vi "uTTA_GetDeviceCalibration.vi"(4 "error in":errorcluster, 7 "VISA Refnum in":refnum<visa-resource-name>) -> (0 "error out":errorcluster, 1 "uTTA_CalData":T1(array[cluster]), 2 "Received":string, 3 "VISA Refnum out":refnum<visa-resource-name>)   [LabVIEW 2021]
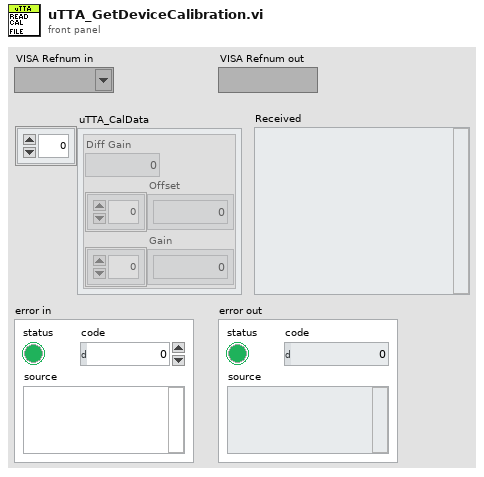
[diagram p1: front panel]
types:
  T1 = cluster{"Diff Gain":dbl, "Offset":dbl[], "Gain":dbl[]}[]
  T2 = cluster{"Diff Gain":dbl, "Offset":dbl[], "Gain":dbl[]}
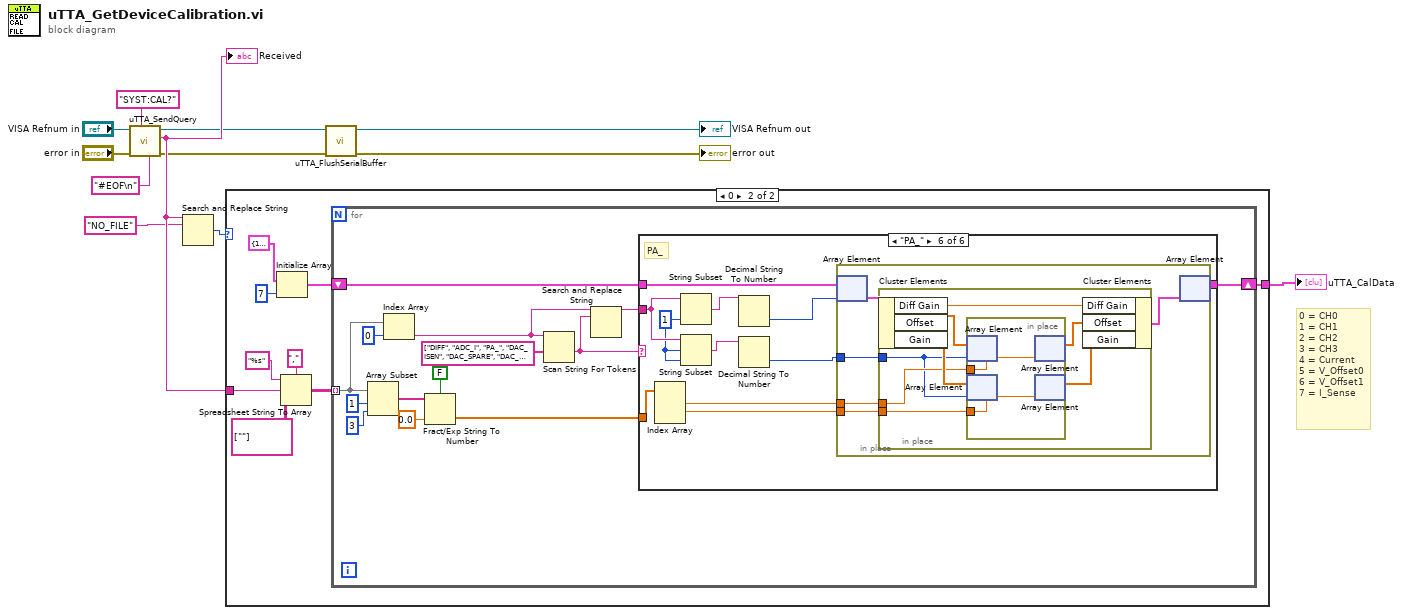
[diagram p0: block diagram]
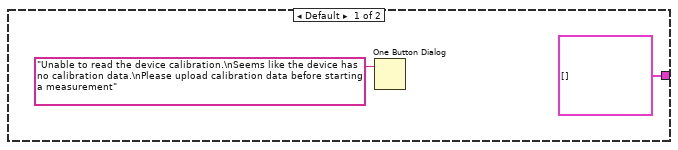
[diagram p2: hidden frame]
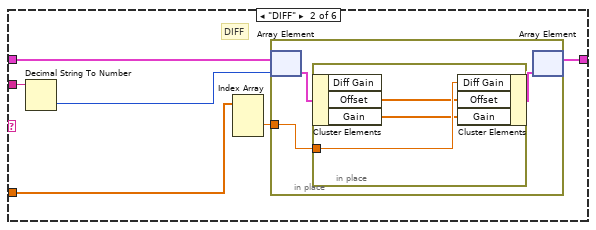
[diagram p4: hidden frame]
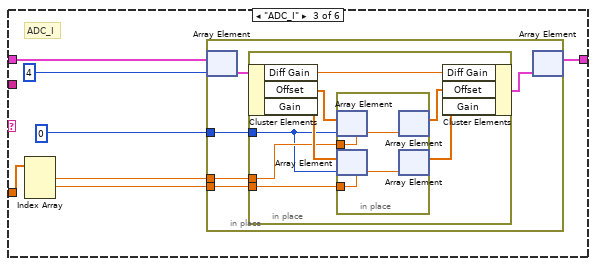
[diagram p5: hidden frame]
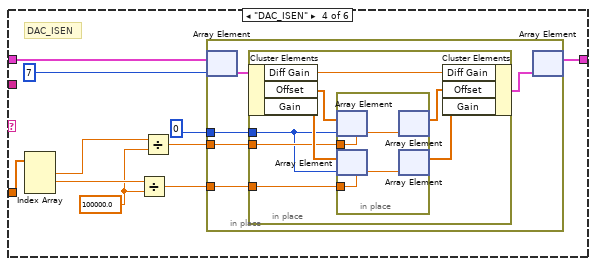
[diagram p6: hidden frame]
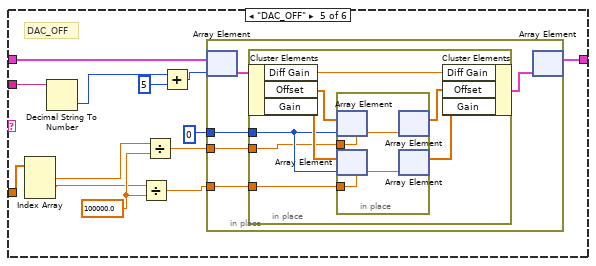
[diagram p7: hidden frame]
diagram:
  # "0 = CH0\n1 = CH1\n2 = CH2\n3 = CH3\n4 = Current\n5 = V_Offset0\n6 = V_Offset1\n7 = I_Sense"
  n1 = call "uTTA_SendQuery.vi"("RX Termination(\\n)"="#EOF\n" ("RX Termination(\\n)"), "Send String"="SYST:CAL?", "error in (no error)"="error in", "VISA Refnum in"="VISA Refnum in") -> ("error out"=w5:errorcluster, "Received"=w8:string, "VISA Refnum out"=w4:refnum<visa-resource-name>)  [unwired: 5 in]
  "Received" <- w8
  n2 = Search and Replace String(input string=w8, search string="NO_FILE") -> (number of replacements=w6:i32)  [unwired: 6 in, 3 out]
  n3 = case shown="0" w6 {
    tunnel: [T1 [] w17] -> w9
    tunnel: w8 -> [_ w16]
    frame Default {
      n4 = One Button Dialog(message="Unable to read the device calibration.\nSeems like the device has no calibration data.\nPlease upload calibration data before starting a measurement") -> ()  [unwired: 1 in, 1 out]
    }
    frame 0 {
      n5 = Initialize Array(T2 {"Diff Gain"=1.0, "Offset"=[0.0, 0.0, 0.0, 0.0], "Gain"=[0.0, 0.0, 0.0, 0.0]} ("Cluster"), 7 ("dimension size")) -> (w18:T1)
      n6 = Spreadsheet String To Array(delimiter (Tab)=",", format string="%s", spreadsheet string=w16, array type (2D Dbl)=string[][] [[""]]) -> (array=w21:string[][])
      n7 = for {
        tunnel: w21 -> [w34] mode=indexing
        shift-right: [w35] -> w17
        shift-left: w18 -> [w36]
        n8 = Array Subset(array=w34, index=1, length=3) -> (w31:string[])
        n9 = Index Array(array=w34, index=0) -> (element=w26:string)
        n10 = Fract/Exp String To Number(use system decimal point (T)=FALSE, string=w31, default (0 dbl)=0.0 ("default (0 DBL)")) -> (number=w28:dbl[])  [unwired: 1 in, 1 out]
        n11 = Scan String For Tokens(7:string[] ["DIFF", "ADC_I", "PA_", "DAC_ISEN", "DAC_SPARE", "DAC_OFF"] ("operators (none)"), 9:w26) -> (1:w25:string)  [unwired: 4 in, 3 out]
        n12 = Search and Replace String(input string=w26, search string=w25) -> (result string=w24:string)  [unwired: 6 in, 3 out]
        n13 = case shown="\"PA_\"" w25 {
          tunnel: w36 -> [w38 w44 w56 w81 w110 w136]
          tunnel: [w38 w43 w55 w80 w109 w135] -> w35
          tunnel: w28 -> [_ w42 w54 w79 w108 w134]
          tunnel: w24 -> [_ w40 _ _ w106 w131]
          frame Default {
          }
          frame "DIFF" {
            # "DIFF"
            n14 = Decimal String To Number(string=w40) -> (number=w39:i32)  [unwired: 2 in, 1 out]
            n15 = Index Array(array=w42) -> (element #2=w41:dbl)  [unwired: 3 in, 2 out]
            n16 = in-place {
              in-place-border: w41 -> [w45]
              n17 = in-place-array #1(w44, w39) -> (w47:T2)
              n18 = in-place {
                in-place-border: w45 -> [w50]
                n19 = in-place-cluster #2(w47) -> ("Offset"=w49:dbl[], "Gain"=w48:dbl[])  [unwired: 1 out]
                n20 = in-place-cluster #2("Diff Gain"=w50, "Offset"=w49, "Gain"=w48) -> (w46:T2)
              }
              n21 = in-place-array #1(w46) -> (w43:T1)  [unwired: 1 out]
            }
          }
          frame "ADC_I" {
            # "ADC_I"
            n22 = Index Array(array=w54) -> (element #1=w52:dbl, element #2=w53:dbl)  [unwired: 3 in, 1 out]
            n23 = in-place {
              in-place-border: w53 -> [w60]
              in-place-border: w52 -> [w59]
              in-place-border: 0 -> [w58]
              n24 = in-place-array #3(w56, 4) -> (w62:T2)
              n25 = in-place {
                in-place-border: w60 -> [w65]
                in-place-border: w59 -> [w66]
                in-place-border: w58 -> [w64]
                n26 = in-place-cluster #4(w62) -> ("Diff Gain"=w63:dbl, "Offset"=w70:dbl[], "Gain"=w69:dbl[])
                n27 = in-place {
                  in-place-border: w66 -> [w72]
                  in-place-border: w65 -> [w71]
                  n28 = in-place-array #5(w70, w64) -> ()  [unwired: 1 out]
                  n29 = in-place-array #6(w69, w64) -> ()  [unwired: 1 out]
                  n30 = in-place-array #5(w72) -> (w68:dbl[])  [unwired: 1 out]
                  n31 = in-place-array #6(w71) -> (w67:dbl[])  [unwired: 1 out]
                }
                n32 = in-place-cluster #4("Diff Gain"=w63, "Offset"=w68, "Gain"=w67) -> (w61:T2)
              }
              n33 = in-place-array #3(w61) -> (w55:T1)  [unwired: 1 out]
            }
          }
          frame "DAC_ISEN" {
            w73 = 100000.0 ("y")
            # "DAC_ISEN"
            n34 = Index Array(array=w79) -> (element #1=w77:dbl, element #2=w75:dbl)  [unwired: 3 in, 1 out]
            n35 = Divide(x=w75, y=w73) -> (x/y=w74:dbl)
            n36 = Divide(x=w77, y=w73) -> (x/y=w76:dbl)
            n37 = in-place {
              in-place-border: w74 -> [w85]
              in-place-border: w76 -> [w84]
              in-place-border: 0 -> [w83]
              n38 = in-place-array #7(w81, 7) -> (w87:T2)
              n39 = in-place {
                in-place-border: w85 -> [w90]
                in-place-border: w84 -> [w91]
                in-place-border: w83 -> [w89]
                n40 = in-place-cluster #8(w87) -> ("Diff Gain"=w88:dbl, "Offset"=w95:dbl[], "Gain"=w94:dbl[])
                n41 = in-place {
                  in-place-border: w91 -> [w97]
                  in-place-border: w90 -> [w96]
                  n42 = in-place-array #9(w95, w89) -> ()  [unwired: 1 out]
                  n43 = in-place-array #10(w94, w89) -> ()  [unwired: 1 out]
                  n44 = in-place-array #9(w97) -> (w93:dbl[])  [unwired: 1 out]
                  n45 = in-place-array #10(w96) -> (w92:dbl[])  [unwired: 1 out]
                }
                n46 = in-place-cluster #8("Diff Gain"=w88, "Offset"=w93, "Gain"=w92) -> (w86:T2)
              }
              n47 = in-place-array #7(w86) -> (w80:T1)  [unwired: 1 out]
            }
          }
          frame "DAC_OFF" {
            w105 = 100000.0 ("y")
            # "DAC_OFF"
            n48 = Index Array(array=w108) -> (element #1=w102:dbl, element #2=w101:dbl)  [unwired: 3 in, 1 out]
            n49 = Decimal String To Number(string=w106) -> (number=w99:i32)  [unwired: 2 in, 1 out]
            n50 = Divide(x=w101, y=w105) -> (x/y=w103:dbl)
            n51 = Divide(x=w102, y=w105) -> (x/y=w104:dbl)
            n52 = Add(x=w99, y=5) -> (x+y=w100:i32)
            n53 = in-place {
              in-place-border: w103 -> [w113]
              in-place-border: 0 -> [w112]
              in-place-border: w104 -> [w111]
              n54 = in-place-array #11(w110, w100) -> (w115:T2)
              n55 = in-place {
                in-place-border: w113 -> [w119]
                in-place-border: w112 -> [w118]
                in-place-border: w111 -> [w116]
                n56 = in-place-cluster #12(w115) -> ("Diff Gain"=w117:dbl, "Offset"=w123:dbl[], "Gain"=w122:dbl[])
                n57 = in-place {
                  in-place-border: w116 -> [w125]
                  in-place-border: w119 -> [w124]
                  n58 = in-place-array #13(w123, w118) -> ()  [unwired: 1 out]
                  n59 = in-place-array #14(w122, w118) -> ()  [unwired: 1 out]
                  n60 = in-place-array #13(w125) -> (w121:dbl[])  [unwired: 1 out]
                  n61 = in-place-array #14(w124) -> (w120:dbl[])  [unwired: 1 out]
                }
                n62 = in-place-cluster #12("Diff Gain"=w117, "Offset"=w121, "Gain"=w120) -> (w114:T2)
              }
              n63 = in-place-array #11(w114) -> (w109:T1)  [unwired: 1 out]
            }
          }
          frame "PA_" {
            w130 = 1 ("length (rest)")
            # "PA_"
            n64 = Index Array(array=w134) -> (element #1=w132:dbl, element #2=w133:dbl)  [unwired: 3 in, 1 out]
            n65 = String Subset(string=w131, length (rest)=w130) -> (substring=w129:string)  [unwired: 1 in]
            n66 = String Subset(string=w131, offset (0)=w130, length (rest)=w130) -> (substring=w128:string)
            n67 = Decimal String To Number(string=w129) -> (number=w127:i32)  [unwired: 2 in, 1 out]
            n68 = Decimal String To Number(string=w128) -> (number=w126:i32)  [unwired: 2 in, 1 out]
            n69 = in-place {
              in-place-border: w133 -> [w139]
              in-place-border: w132 -> [w138]
              in-place-border: w126 -> [w137]
              n70 = in-place-array #15(w136, w127) -> (w141:T2)
              n71 = in-place {
                in-place-border: w139 -> [w144]
                in-place-border: w138 -> [w145]
                in-place-border: w137 -> [w143]
                n72 = in-place-cluster #16(w141) -> ("Diff Gain"=w142:dbl, "Offset"=w149:dbl[], "Gain"=w148:dbl[])
                n73 = in-place {
                  in-place-border: w145 -> [w151]
                  in-place-border: w144 -> [w150]
                  n74 = in-place-array #17(w149, w143) -> ()  [unwired: 1 out]
                  n75 = in-place-array #18(w148, w143) -> ()  [unwired: 1 out]
                  n76 = in-place-array #17(w151) -> (w147:dbl[])  [unwired: 1 out]
                  n77 = in-place-array #18(w150) -> (w146:dbl[])  [unwired: 1 out]
                }
                n78 = in-place-cluster #16("Diff Gain"=w142, "Offset"=w147, "Gain"=w146) -> (w140:T2)
              }
              n79 = in-place-array #15(w140) -> (w135:T1)  [unwired: 1 out]
            }
          }
        }
      }
    }
  }
  "uTTA_CalData" <- w9
  n80 = call "uTTA_FlushSerialBuffer.vi"("error in (no error)"=w5, "VISA Refnum in"=w4) -> ("error out"=→"error out":errorcluster, "VISA Refnum out"=→"VISA Refnum out":refnum<visa-resource-name>)  [unwired: 4 in]
